vi "SetStepResults.vi"(8 "Multiple Numeric Limit Test Results":dbl[](array[numeric])=[1.0, 2.0, 3.0], 9 "Pass/Fail 1 Result":bool=TRUE, 10 "Pass/Fail 2 Result":bool, 11 "Sequence Context In":refnum<k7>) -> (0 "error out":errorcluster)   [LabVIEW 2011]
doc: "This VI demonstrates how to cast a SequenceFile object in order access properties of the PropertyObjectFile and PropertyObject parent classes"
uses:
  <vilib>/addons/TestStand/_TSUtility.llb/TestStand - Set Property Value (Boolean).vi
  <vilib>/addons/TestStand/_TSUtility.llb/TestStand - Set Property Value (Numeric Array).vi
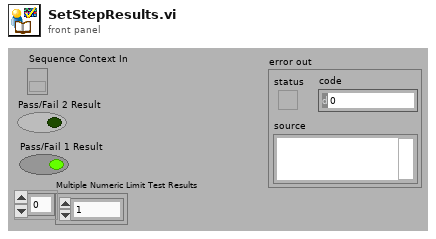
[diagram p1: front panel]
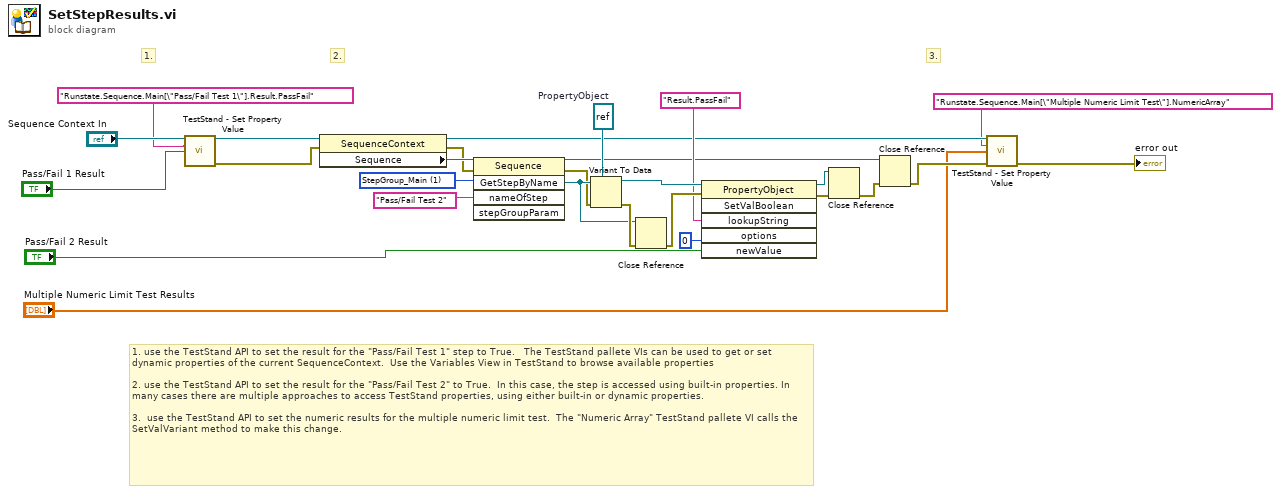
[diagram p0: block diagram]
diagram:
  w16 = 1 items=["StepGroup_Setup", "StepGroup_Main", "StepGroup_Cleanup"] ("stepGroupParam")
  w22 = refnum<k7> refnum  # PropertyObject
  # "3."
  # "2."
  # "1."
  # "1. use the TestStand API to set the result for the \"Pass/Fail Test 1\" step to True.   The TestStand pallete VIs can be used to get or set dynamic properties of the current SequenceContext.  Use the Variables View in TestStand to browse available properties\n\n2. use the TestStand API to set the result for the \"Pass/Fail Test 2\" to True.  In this case, the step is accessed using built-in properties. In many cases there are multiple approaches to access TestStand properties, using either built-in or dynamic properties.\n\n3.  use the TestStand API to set the numeric results for the multiple numeric limit test.  The \"Numeric Array\" TestStand pallete VI calls the SetValVariant method to make this change."
  n1 = call-poly <vilib>:"TestStand - Set Property Value.vi"("Sequence Context In"="Sequence Context In", "Lookup String"="Runstate.Sequence.Main[\"Pass/Fail Test 1\"].Result.PassFail", "New Value"="Pass/Fail 1 Result") -> ("Sequence Context Out"=w9:refnum<k7>, "error out"=w8:errorcluster)  [unwired: 11 in]
  n2 = property class="SequenceContext"(reference=w9, error in=w8) -> (reference out=w5:refnum<k7>, error out=w15:errorcluster, "Sequence"=w24:refnum<k7>)
  n3 = invoke class="Sequence" method="GetStepByName"(reference=w24, error in=w15, "nameOfStep"="Pass/Fail Test 2", "stepGroupParam"=w16) -> (reference out=w12:refnum<k7>, error out=w7:errorcluster, "GetStepByName"=w20:refnum<k7>)  [unwired: 1 in, 2 out]
  n4 = Variant To Data(error in=w7, type=w22, Variant=w20) -> (data=w19:refnum<k7>, error out=w21:errorcluster)
  n5 = Close Reference(reference=w20, error in (no error)=w21) -> (error out=w18:errorcluster)
  n6 = invoke class="PropertyObject" method="SetValBoolean"(reference=w19, error in=w18, "lookupString"="Result.PassFail" ("Lookup String"), "options"=0, "newValue"="Pass/Fail 2 Result") -> (reference out=w14:refnum<k7>, error out=w13:errorcluster)  [unwired: 1 in, 4 out]
  n7 = Close Reference(reference=w14, error in (no error)=w13) -> (error out=w11:errorcluster)
  n8 = Close Reference(reference=w12, error in (no error)=w11) -> (error out=w4:errorcluster)
  n9 = call-poly <vilib>:"TestStand - Set Property Value.vi"("Sequence Context In"=w5, "Lookup String"="Runstate.Sequence.Main[\"Multiple Numeric Limit Test\"].NumericArray", "New Value"="Multiple Numeric Limit Test Results", "error in (no error)"=w4) -> ("error out"=→"error out":errorcluster)  [unwired: 10 in, 1 out]
